vi "add.vi"(0 "HB_Simple in":refnum<class "HB_Simple.lvclass">, 2 "y":dbl, 5 "error in (no error)":errorcluster) -> (14 "HB_Simple out":refnum<class "HB_Simple.lvclass">, 19 "error out":errorcluster)   [LabVIEW 2009, in "HB_BaseClass_Examples.lvlib" / "HB_Simple.lvclass"]
doc: "Increment value of x."
uses:
  HB_Simple.lvclass
  HB_Simple.lvclass/HB_Simple.ctl
  lib.lib/HGF_LVC/HGF_BaseClasses/HGF_TriggeredEvent/HGF_TriggeredEvent.lvclass
  lib.lib/HGF_LVC/HGF_BaseClasses/HGF_PVPublisher/HGF_PVPublisher.lvclass
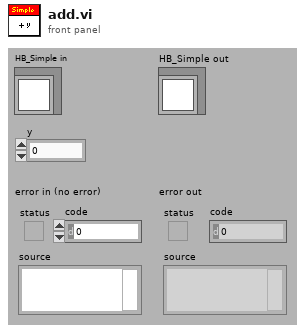
[diagram p1: front panel]
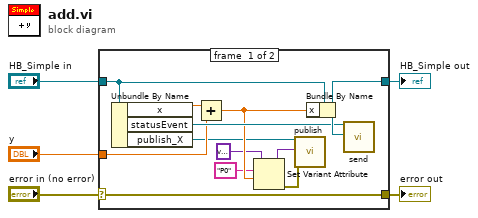
[diagram p0: block diagram]
diagram:
  n1 = case shown="No Error" "error in (no error)" {
    selector: "error in (no error)" -> [w17 w19]
    tunnel: [w17 w19] -> w4
    tunnel: [w16 w18] -> w2
    tunnel: "HB_Simple in" -> [w15 w18]
    tunnel: "y" -> [w12 _]
    frame #0 {
      n2 = Unbundle By Name(w15) -> ("x"=w13:dbl, "statusEvent"=w14:refnum<class "HGF_TriggeredEvent.lvclass">, "publish_X"=w6:refnum<class "HGF_PVPublisher.lvclass">)
      n3 = Add(x=w13, y=w12) -> (x+y=w9:dbl)
      n4 = Set Variant Attribute(Variant=variant ("variant"), name="P0", value=w9) -> (Variant out=w10:variant, error out=w11:errorcluster)  [unwired: 1 in, 1 out]
      n5 = call-dynamic "publish.vi"("HGF_PVPublisher"=w6, "data"=w10, "error in (no error)"=w11) -> ()  [unwired: 2 in, 15 out]
      n6 = Bundle By Name(cluster=w15, "x"=w9) -> (w16:refnum<class "HB_Simple.lvclass">)
      n7 = call-dynamic "send.vi"("HGF_Event"=w14, "Object"=w16) -> ()  [unwired: 3 in, 15 out]
    }
    frame #1 {
    }
  }
  "error out" <- w4
  "HB_Simple out" <- w2
